vi "AcqPtEtalonnageUSB.vi"(4 "entrée d'erreur":errorcluster caption="entrée d'erreur (pas d'erreur)", 7 "Projet":string) -> (0 "sortie d'erreur":errorcluster)   [LabVIEW 2017]
uses:
  DefDeType/WhichPath.ctl
  <vilib>/DAQmx/read.llb/DAQmx Read (Analog 2D DBL NChan NSamp).vi
  <vilib>/DAQmx/miscellaneous.llb/DAQmx Fill In Error Info.vi
  <vilib>/Analysis/NI_AALBase.lvlib
panel:
  out "Graphe 2":dbl[][](graph)
  out "chaîne de type tableur":string
  out "fichier :":path
  out "Glissière":i32(slide) scale=0.0..30.0
  out "tableau ajouté":dbl[](array[numeric]) format="%#.5f"
  out "Ecart-type":dbl[](array[numeric])
  out "Moy":dbl[](array[numeric]) format="%#.5f"
  # "Acquisition d'un point d'étalonnage"
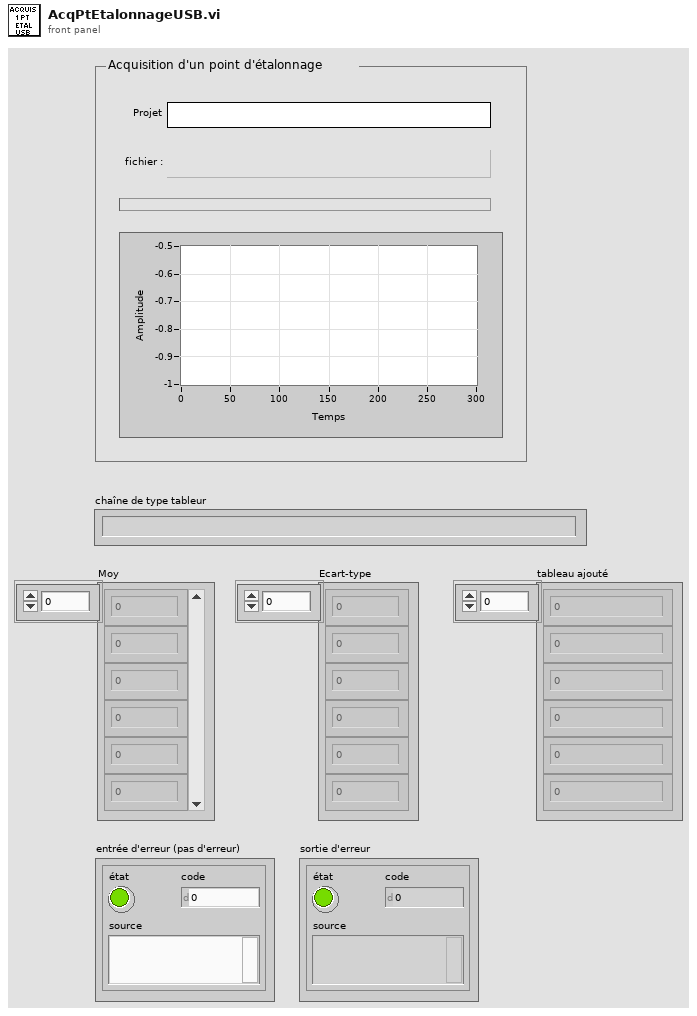
[diagram p1: front panel]
types:
  T1 = typedef "WhichPath.ctl" = enum16{"DossierProjet", "Config", "Meas", "MeasPCI", "MeasCRIO1", "MeasCRIO2", "MeasQualisys", "MeasHBM", "MeasTDMS", "Fig", "Res"}
  T2 = enum16{"open", "replace", "create", "open or create", "replace or create", "replace or create with confirmation"}
  T3 = typedef "ConfigTotale.ctl" = cluster{"VoltageChannels":T4, "WheastoneBridgeChannels":T5, "Configuration":T6}
  T4 = typedef "VoltageChannels.ctl" = cluster{"ChannelNames":string[], "Sensitivity(Unit/V)":dbl[], "AutoZero":bool[], "ChannelUnits":string[], "Offsets(Units)":dbl[], "Graph Num":u8[]}
  T5 = typedef "WBridgeChannels.ctl" = cluster{"ChannelNames":string[], "Sensitivity(Unit/V)":dbl[], "AutoZero":bool[], "ChannelUnits":string[], "Offsets(Units)":dbl[], "Graph Num":u8[]}
  T6 = typedef "Configuration.ctl" = cluster{"AcqSamplingRate(Hz)":u32, "AcqTime(s)":u32, "Trigger":bool, "NbVoltageChannels":u32, "NbWBridgeChannels":u32, "Qualisys":bool, "Hexapode":bool, "FinalSamplingRate(Hz)":u32, "QualisysDataType":enum16{"6DOF", "3DTracking", "6DOF + 3D"}, "Nortek":bool, "HBM":bool}
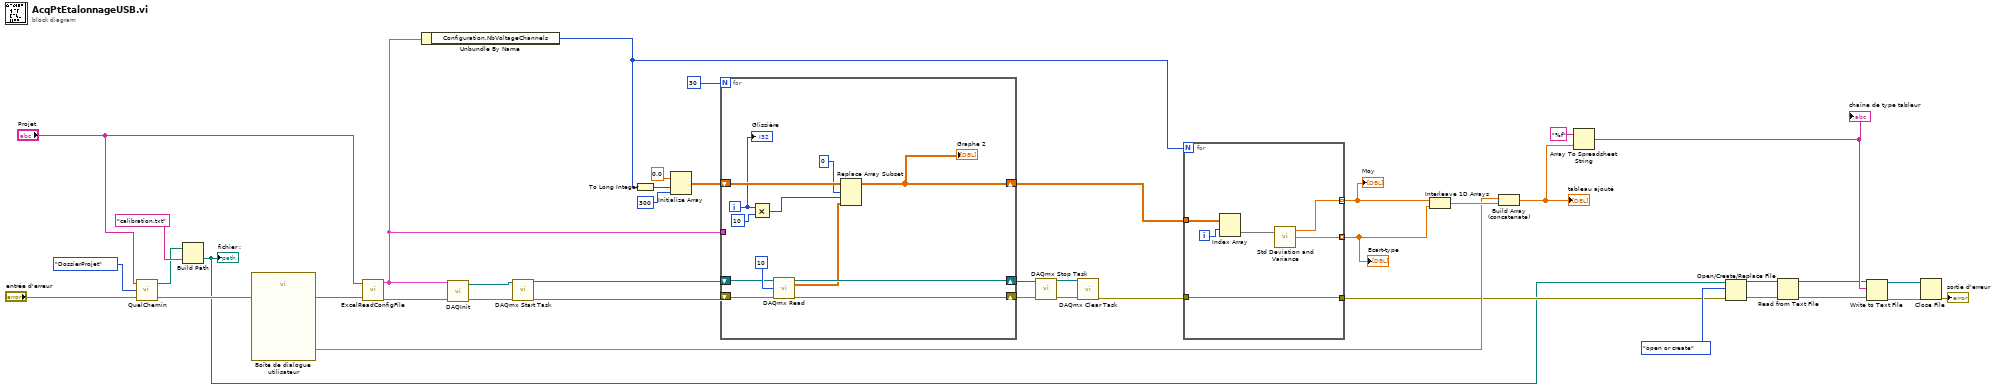
[diagram p0: block diagram]
diagram:
  n1 = call "QuelChemin.vi"("Entrée d'erreur"="entrée d'erreur", "WhichPath?"=WhichPath."DossierProjet", "NomProjet"="Projet") -> ("Sortie d'erreur"=w20:errorcluster, "SurDisqueLocal"=w17:path)  [unwired: 1 out]
  n2 = Build Path(base path=w17, name or relative path="calibration.txt" ("nom ou chemin relatif")) -> (appended path=w16:path)
  "fichier :" <- w16
  n3 = call "Boîte de dialogue utilisateur"("error in (no error)"=w20) -> ("ValRef"=w35:dbl, "error out"=w39:errorcluster)  [unwired: 16 in, 1 out]
  n4 = call "ExcelReadConfigFile.vi"("NomProjet"="Projet", "error in (no error)"=w39) -> ("ConfigurationTotale"=w13:T3, "error out"=w15:errorcluster)  [unwired: 3 in]
  n5 = Unbundle By Name(w13) -> ("Configuration.NbVoltageChannels"=w3:u32)
  n6 = call "DAQInit.vi"("error in"=w15, "configInput"=w13) -> ("error out"=w14:errorcluster, "task out"=w12:refnum<k21>)  [unwired: 2 in]
  n7 = call <vilib>:"DAQmx Start Task.vi"("task/channels in"=w12, "error in"=w14) -> ("task out"=w10:refnum<k21>, "error out"=w11:errorcluster)  [unwired: 12 in]
  n8 = To Long Integer(number=w3) -> (32bit integer=w4:i32)
  n9 = Initialize Array(0.0 ("élément"), w4, 300 ("taille de la dimension")) -> (w41:dbl[][])
  n10 = for {
    N: 30 ("taille de la dimension") -> [_]
    shift-right: [w49] -> w8
    shift-left: w11 -> [w53]
    shift-right: [w43] -> w1
    shift-left: w41 -> [w54]
    tunnel: w13 -> [_]
    shift-right: [w50] -> w9
    shift-left: w10 -> [w51]
    i -> [w47]
    n11 = Multiply(x=w47, y=10) -> (x*y=w44:i32)
    n12 = call-poly <vilib>:"DAQmx Read.vi"("task/channels in"=w51, "number of samples per channel"=10, "error in"=w53) -> ("task out"=w50:refnum<k21>, "data"=w46:dbl[][], "error out"=w49:errorcluster)  [unwired: 10 in]
    n13 = Replace Array Subset(array=w54, new element=w46, index (row)=0 ("indice désactivé (col)"), index (col)=w44) -> (w43:dbl[][])
    "Graphe 2" <- w43
    "Glissière" <- w47
  }
  n14 = call <vilib>:"DAQmx Stop Task.vi"("task/channels in"=w9, "error in"=w8) -> ("task out"=w6:refnum<k21>, "error out"=w7:errorcluster)  [unwired: 12 in]
  n15 = call <vilib>:"DAQmx Clear Task.vi"("task in"=w6, "error in"=w7) -> ("error out"=w5:errorcluster)  [unwired: 13 in]
  n16 = for {
    N: w3 -> [_]
    tunnel: w5 -> [w60]
    tunnel: [w60] -> w23
    tunnel: [w59] -> w38 mode=indexing
    tunnel: [w58] -> w37 mode=indexing
    tunnel: w1 -> [w57]
    i -> [w56]
    n17 = Index Array(array=w57, index (row)=w56) -> (element=w55:dbl[])  [unwired: 1 in]
    n18 = call <vilib>:"Std Deviation and Variance.vi"("X"=w55) -> ("mean"=w59:dbl, "standard deviation"=w58:dbl)  [unwired: 1 in, 1 out]
  }
  "Moy" <- w38
  "Ecart-type" <- w37
  n19 = Interleave 1D Arrays(w38, w37) -> (w36:dbl[])
  n20 = Build Array (concatenate)(w35, w36) -> (w33:dbl[])
  "tableau ajouté" <- w33
  n21 = Array To Spreadsheet String(array=w33, 3:"%f" ("chaîne de format")) -> (spreadsheet string=w29:string)  [unwired: 1 in]
  "chaîne de type tableur" <- w29
  n22 = Open/Create/Replace File(file path (use dialog)=w16, error in=w23, operation (0:open)=T2."open or create" ("opération (0 : open)")) -> (refnum out=w26:refnum<file>, error out=w25:errorcluster)  [unwired: 3 in, 1 out]
  n23 = Read from Text File(file (use dialog)=w26, error in=w25) -> (refnum out=w27:refnum<file>, error out=w28:errorcluster)  [unwired: 2 in, 2 out]
  n24 = Write to Text File(file (use dialog)=w27, text=w29, error in=w28) -> (refnum out=w30:refnum<file>, error out=w31:errorcluster)  [unwired: 1 in, 1 out]
  n25 = Close File(refnum=w30, error in=w31) -> (error out=→"sortie d'erreur":errorcluster)  [unwired: 1 out]
